vi "Construct.vi"(8 "error in (no error)":errorcluster, 10 "hardware config file":path=path "c:/ni-rt/VeriStand/Custom Devices/Ballard/MIL-STD-1553/1553_HW_Reference_007.xml", 11 "device parameters":T1) -> (0 "error out":errorcluster, 3 "Ballard 1553 shared resources":refnum<class "Shared Resources.lvclass">)   [LabVIEW 2020, in "Ballard MIL-STD-1553 Engine.lvlib" / "Implementation.lvlib" / "Shared Resources.lvclass"]
uses:
  Shared Resources.lvclass
  Shared/Device Parameters.ctl
  Shared/Initialization Method.ctl
  Shared Resources.lvclass/Shared Resources.ctl
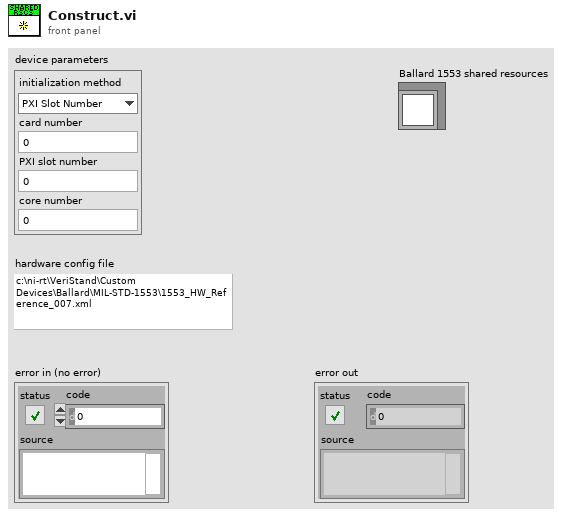
[diagram p1: front panel]
types:
  T1 = typedef "Device Parameters.ctl" = cluster{"initialization method":T2, "card number":i32, "PXI slot number":i32, "core number":i32}
  T2 = typedef "Initialization Method.ctl" = enum16{"PXI Slot Number", "Card Number"}
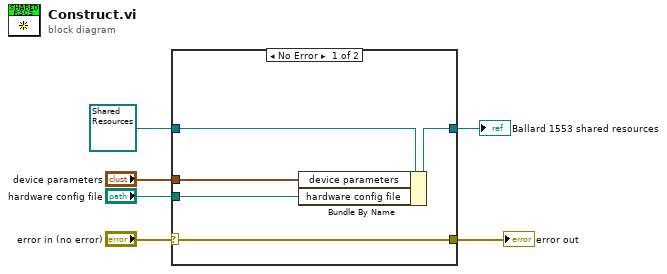
[diagram p0: block diagram]
diagram:
  n1 = case shown="No Error" "error in (no error)" {
    selector: "error in (no error)" -> [w9 w12]
    tunnel: refnum<class "Shared Resources.lvclass"> refnum ("Communication Bus Template Interfaces:Implementation.lvlib:Shared Resources.lvclass") -> [w11 w13]
    tunnel: [w10 w13] -> w5
    tunnel: [w9 w12] -> w3
    tunnel: "hardware config file" -> [w8 _]
    tunnel: "device parameters" -> [w7 _]
    frame No Error {
      n2 = Bundle By Name(cluster=w11, "device parameters"=w7, "hardware config file"=w8) -> (w10:refnum<class "Shared Resources.lvclass">)
    }
    frame Error {
    }
  }
  "error out" <- w3
  "Ballard 1553 shared resources" <- w5
